vi "header.vi"(3 "error in":errorcluster, 5 "TCP Network Connection in":refnum<k5>) -> (0 "error out":errorcluster, 1 "Sensor sample":T1, 2 "TCP Network Connection out":refnum<k5>)   [LabVIEW 2019, in "Lib_Simx.lvlib"]
doc: "Parse data from sensor into a cluster given a connection ID."
uses:
  Lib_Simx.lvlib
  controls/sensor_sample.ctl
  controls/Header.ctl
panel:
  in  "frame_count":u32
  in  "game_time":u32
  in  "time_stamp":u32
  in  "length":u32
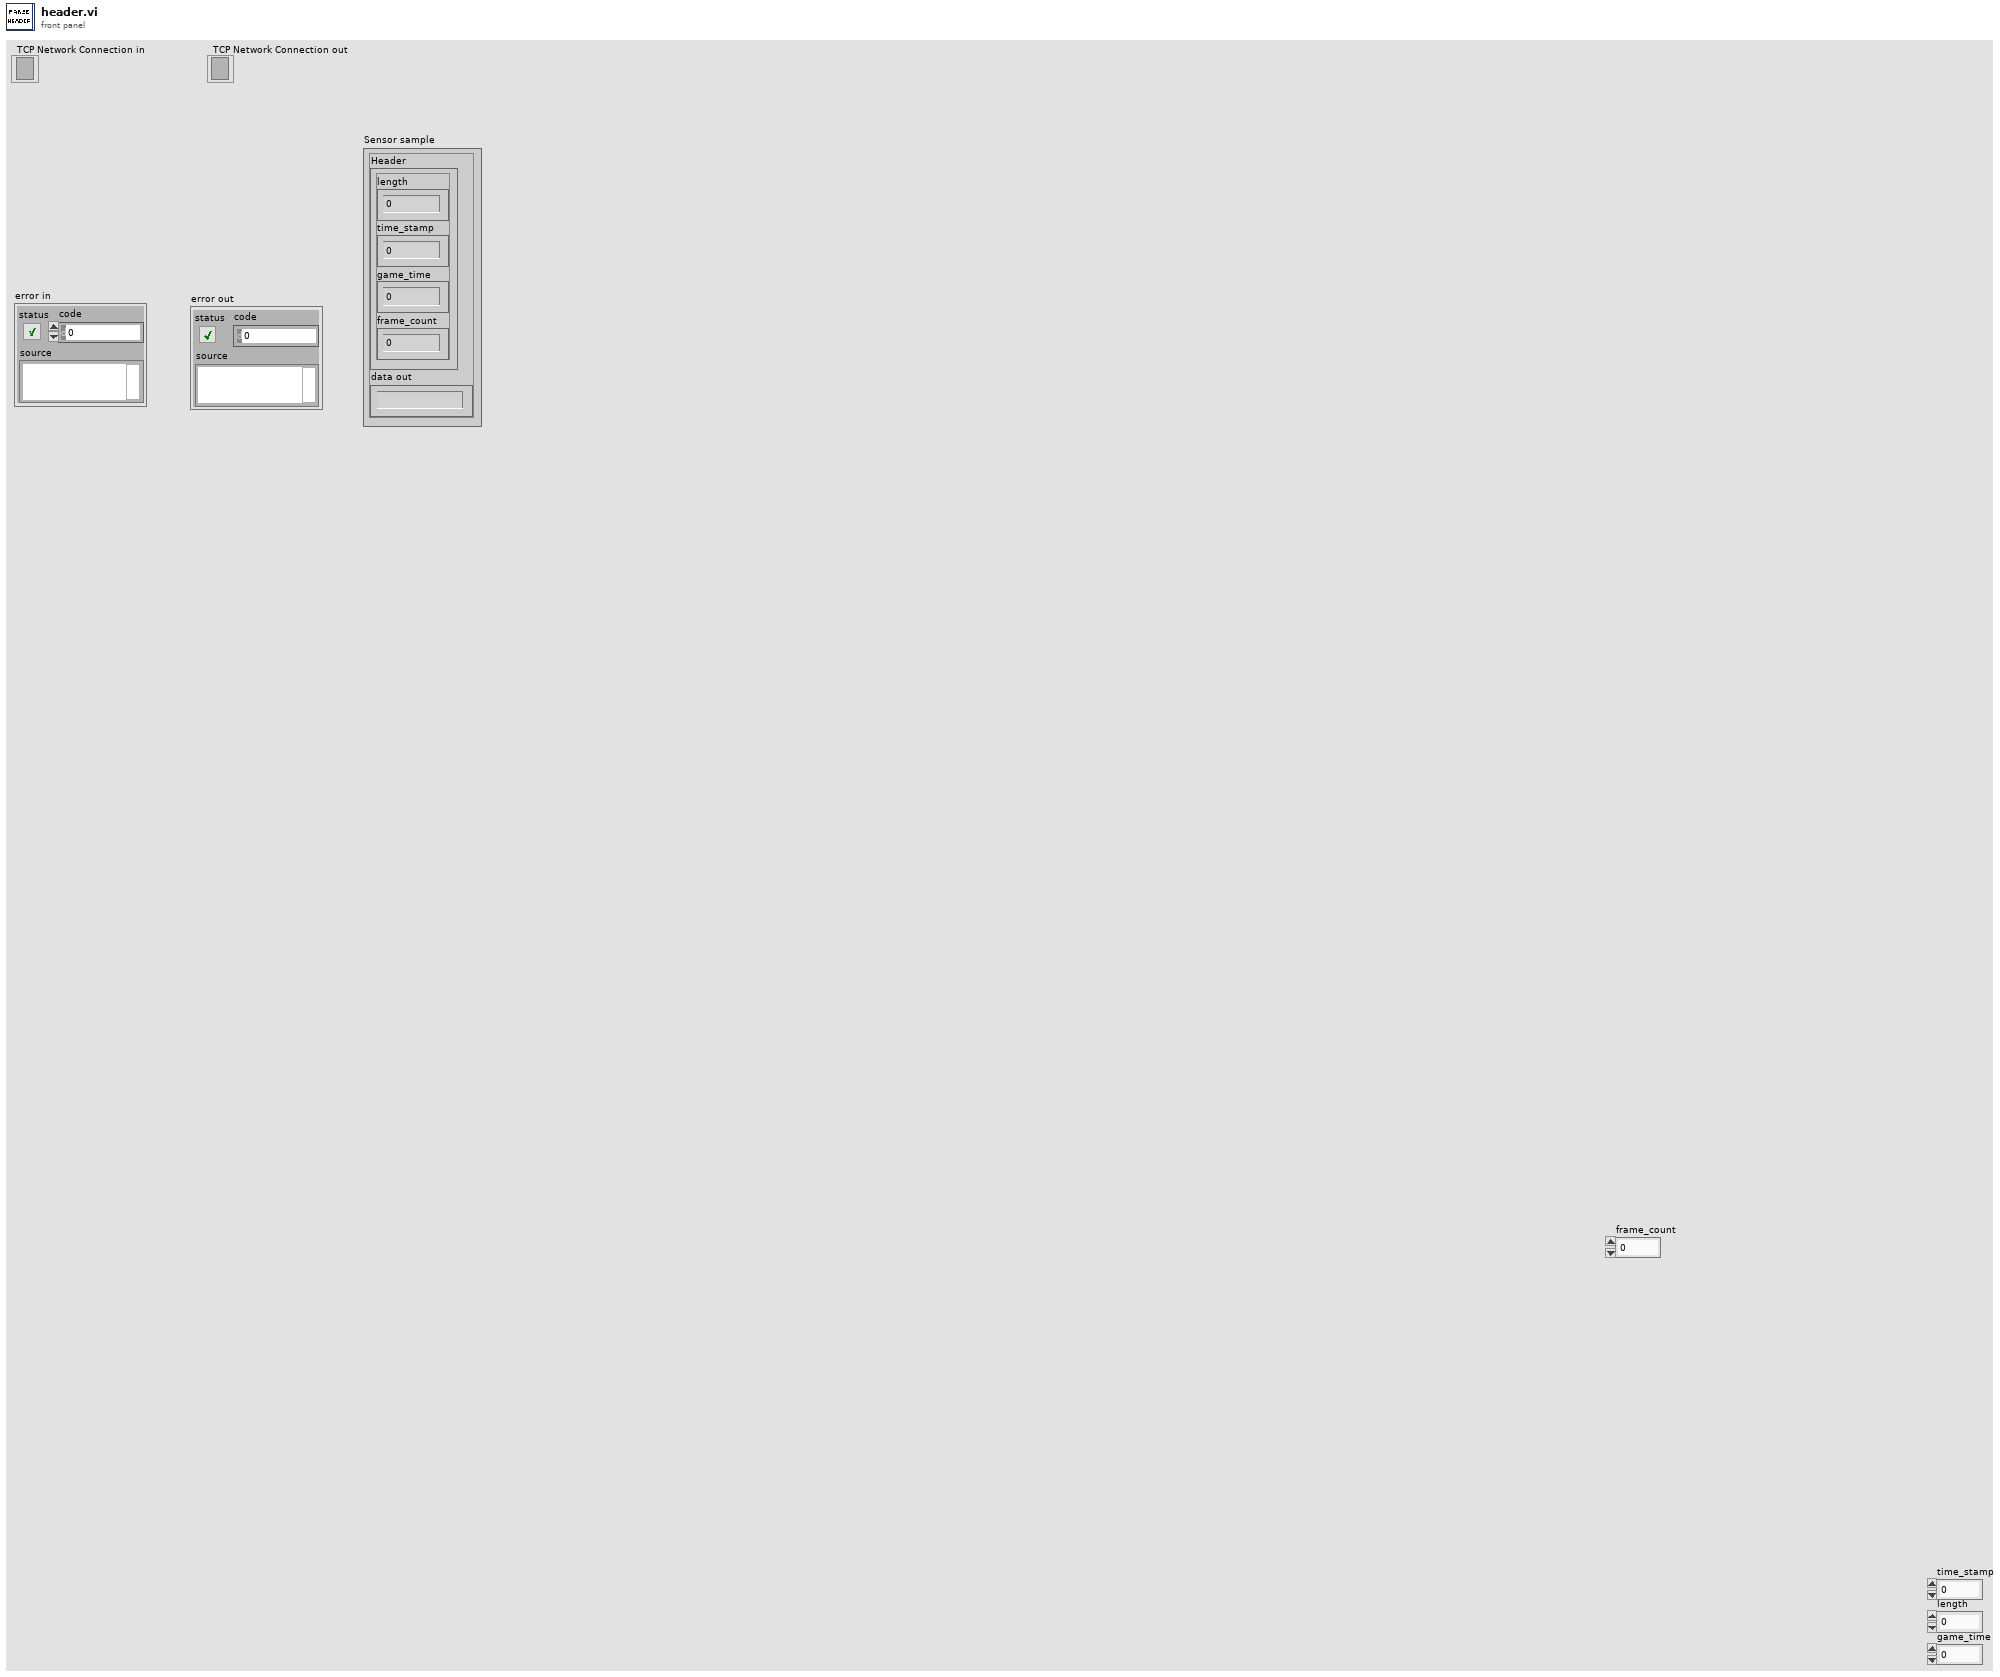
[diagram p1: front panel]
types:
  T1 = typedef "Lib_Simx.lvlib/sensor_sample.ctl" = cluster{"Header":T2, "data out":string}
  T2 = typedef "Lib_Simx.lvlib/Header.ctl" = cluster{"length":u32, "time_stamp":u32, "game_time":sgl, "frame_count":u32}
  T3 = enum16{"big-endian, network order", "native, host order", "little-endian"}
  T4 = cluster{"length":u32, "time_stamp":u32, "game_time":u32, "frame_count":u32}
  T5 = cluster{cluster{"length":u32, "time_stamp":u32, "game_time":u32, "frame_count":u32}, "data out":string}
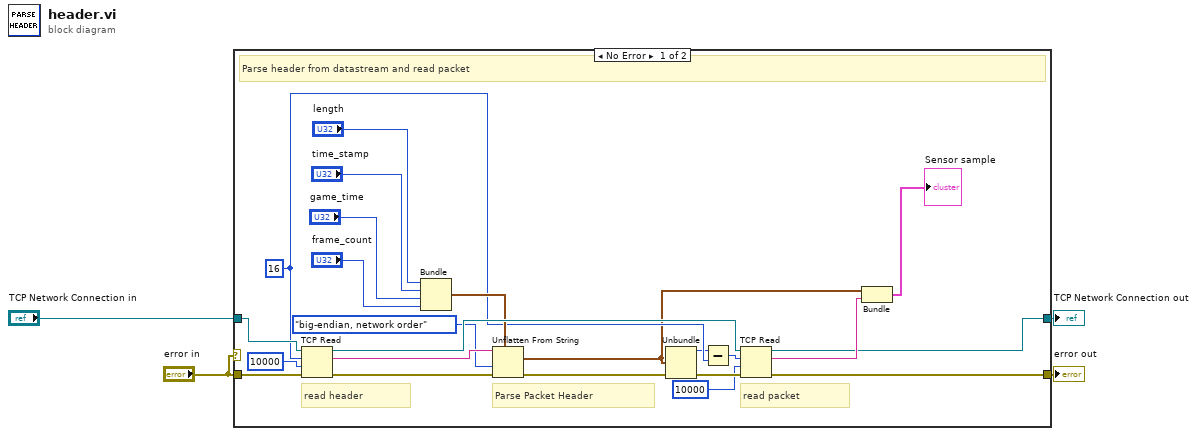
[diagram p0: block diagram]
diagram:
  n1 = case shown="No Error" "error in" {
    tunnel: "error in" -> [w12 w27]
    tunnel: "TCP Network Connection in" -> [w19 w28]
    tunnel: [w16 w28] -> w3
    tunnel: [w15 w27] -> w2
    frame No Error {
      w13 = 16 ("bytes to read")
      # "read packet"
      # "read header"
      # "Parse Packet Header"
      # "Parse header from datastream and read packet"
      n2 = TCP Read(connection ID=w19, bytes to read=w13, error in (no error)=w12, 9:10000 ("timeout ms (25000)")) -> (connection ID out=w23:refnum<k5>, data out=w24:string, error out=w25:errorcluster)  [unwired: 1 in]
      n3 = Bundle("length"="length", "time_stamp"="time_stamp", "game_time"="game_time", "frame_count"="frame_count") -> (w18:T4)  [unwired: 1 in]
      n4 = Unflatten From String(type=w18, binary string=w24, byte order (0:big-endian, network order)=T3."big-endian, network order", error in (no error)=w25) -> (value=w9:T4, error out=w26:errorcluster)  [unwired: 1 in, 1 out]
      n5 = Unbundle(w9) -> ("length"=w5:u32)  [unwired: 3 out]
      n6 = Subtract(x=w5, y=w13) -> (x-y=w11:u32)
      n7 = TCP Read(connection ID=w23, bytes to read=w11, error in (no error)=w26, 9:10000 ("timeout ms (25000)")) -> (connection ID out=w16:refnum<k5>, data out=w17:string, error out=w15:errorcluster)  [unwired: 1 in]
      n8 = Bundle(w9, "data out"=w17) -> (→"Sensor sample":T5)  [unwired: 1 in]
    }
    frame Error {
    }
  }
  "TCP Network Connection out" <- w3
  "error out" <- w2
